vi "HTTPResponseHeaderLine.vi"(8 "error in (no error)":errorcluster, 11 "HTTP Request Line":string) -> (0 "error out":errorcluster, 1 "Reason-Phrase":string, 2 "Status Code":T1=101 items=["Switching Protocols"=101, "Bad Request"=400, "Forbidden"=403, "Not Found"=404, "Upgrade Required"=426], 3 "Http Version":string)   [LabVIEW 2016, in "WebSockets.lvlib"]
doc: "Parses the first line of the received HTTP response\nWebSockets 1.6.0.22\nSam Sharp - MediaMongrels Ltd\nCopyright (c) 2016, MediaMongrels Ltd"
uses:
  WebSockets/WebSockets.lvlib
  WebSockets/HTTPResponseCodes.ctl
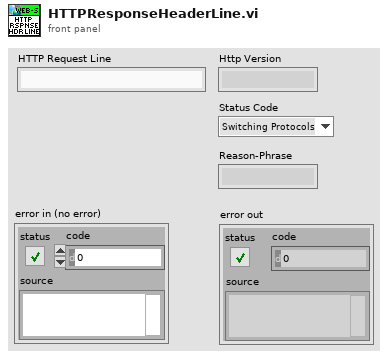
[diagram p1: front panel]
types:
  T1 = typedef "WebSockets.lvlib/HTTPResponseCodes.ctl" = u16
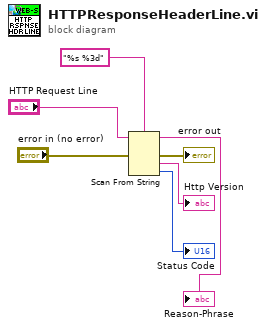
[diagram p0: block diagram]
diagram:
  n1 = Scan From String(format string="%s %3d", input string="HTTP Request Line", error in="error in (no error)") -> (remaining string=→"Reason-Phrase":string, error out=→"error out":errorcluster, output 1=→"Http Version":string, output 2=→"Status Code":T1)  [unwired: 3 in, 1 out]
